vi "test_serialize_deserialize.vi"   [LabVIEW 2020, in "Optitrack.lvlib"]
doc: "Version 0.1"
uses:
  <vilib>/ADAS Record/CustomDataTypes/Optitrack/Optitrack.lvlib
  <vilib>/addons/_JKI Toolkits/Caraya/classes/Test/Test.lvclass
  <vilib>/addons/_JKI Toolkits/Caraya/classes/Assert/Assert.lvclass
  <vilib>/ADAS Record/CustomDataTypes/Optitrack/Process Data.ctl
  <vilib>/ADAS Record/CustomDataTypes/ADAS Generic/Serialize Data.vi
  <vilib>/ADAS Record/CustomDataTypes/ADAS Generic/NI_ADAS_Generic.lvlib
  <vilib>/ADAS Record/CustomDataTypes/ADAS Generic/Deserialize Data.vi
  Projects/NI AzDO/Mercedes-MPIC-201077/Record_MPIC3/mercedes-record-mpic3-201077/software-record-plugins/labview-2020/src/shared/TypeDef-Optitrack-RigidBody.ctl
  Projects/NI AzDO/Mercedes-MPIC-201077/Record_MPIC3/mercedes-record-mpic3-201077/software-record-plugins/labview-2020/src/shared/TypeDef-Optitrack-MarkerPoint.ctl
  Projects/NI AzDO/Mercedes-MPIC-201077/Record_MPIC3/mercedes-record-mpic3-201077/software-record-plugins/labview-2020/src/shared/TypeDef-Optitrack-MarkerSet.ctl
  Projects/NI AzDO/Mercedes-MPIC-201077/Record_MPIC3/mercedes-record-mpic3-201077/software-record-plugins/labview-2020/src/shared/TypeDef-Optitrack-LabeledMarker.ctl
  Projects/NI AzDO/Mercedes-MPIC-201077/Record_MPIC3/mercedes-record-mpic3-201077/software-record-plugins/labview-2020/src/shared/TypeDef-Optitrack-TrackedData.ctl
  Projects/NI AzDO/Mercedes-MPIC-201077/Record_MPIC3/mercedes-record-mpic3-201077/software-record-plugins/labview-2020/src/shared/TypeDef-Optitrack-FrameData.ctl
types:
  T1 = typedef "Optitrack.lvlib/Process Data.ctl" = cluster{"OptitrackFrame":T2}
  T2 = typedef "TypeDef-Optitrack-FrameData.ctl" = cluster{"# Labeled Markers":i32, "Frame":i32, "# Marker Sets":i32, "Relative Timestamp":dbl, "# Other Markers":i32, "# Rigid Bodies":i32, "# Skeletons":i32, "# Force Plates":i32, "# Devices":i32, "Timecode":u32, "Timecode Subframe":u32, "Mid Exposure Timestamp":u64, "Data Received Timestamp":u64, "Transmit Timestamp":u64, "Tracking Models Changed":bool, "Recording":bool, "Tracked Data":T3, "Statistics":cluster{"Dropped Frames":i32, "Frames Remaining":i32, "FPS":dbl}, "Frame Timestamp":timestamp}
  T3 = typedef "TypeDef-Optitrack-TrackedData.ctl" = cluster{"Labled Markers Data":T4[], "Marker Sets Data":T5[], "Rigid Bodies Data":T7[]}
  T4 = typedef "TypeDef-Optitrack-LabeledMarker.ctl" = cluster{"X":sgl, "Y":sgl, "Z":sgl, "Size":sgl, "Residual":sgl, "Parameters":i16, "ID":i32}
  T5 = typedef "TypeDef-Optitrack-MarkerSet.ctl" = cluster{"Marker Set Name":string, "Marker Points":T6[]}
  T6 = typedef "TypeDef-Optitrack-MarkerPoint.ctl" = cluster{"X":sgl, "Y":sgl, "Z":sgl}
  T7 = typedef "TypeDef-Optitrack-RigidBody.ctl" = cluster{"ID":i32, "Mean Error":sgl, "qw":sgl, "qx":sgl, "qy":sgl, "qz":sgl, "Tracked":bool, "x":sgl, "y":sgl, "z":sgl, "Rigid Body Name":string}
  T8 = typedef "NI_ADAS_Generic.lvlib/Process Data.ctl" = cluster{"Timestamp":timestamp, "Bus Channel":u16, "Byte Array":u8[]}
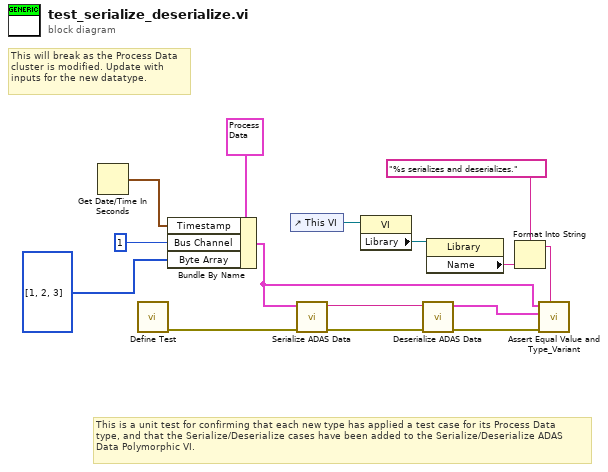
[diagram p0: block diagram]
diagram:
  # "This will break as the Process Data\ncluster is modified. Update with\ninputs for the new datatype."
  # "This is a unit test for confirming that each new type has applied a test case for its Process Data\ntype, and that the Serialize/Deserialize cases have been added to the Serialize/Deserialize ADAS\nData Polymorphic VI."
  n1 = Get Date/Time In Seconds() -> (seconds since 1Jan1904=w4:timestamp)
  n2 = call <vilib>:"Define Test.vi"() -> ("error out"=w10:errorcluster)  [unwired: 11 in]
  n3 = Bundle By Name(cluster=T1 {"OptitrackFrame"={"# Labeled Markers"=0, "Frame"=0, "# Marker Sets"=0, "Relative Timestamp"=0.0, "# Other Markers"=0, "# Rigid Bodies"=0, "# Skeletons"=0, "# Force Plates"=0, "# Devices"=0, "Timecode"=0, "Timecode Subframe"=0, "Mid Exposure Timestamp"=0, "Data Received Timestamp"=0, "Transmit Timestamp"=0, "Tracking Models Changed"=FALSE, "Recording"=FALSE, "Tracked Data"={"Labled Markers Data"=[], "Marker Sets Data"=[], "Rigid Bodies Data"=[]}, "Statistics"={"Dropped Frames"=0, "Frames Remaining"=0, "FPS"=0.0}, "Frame Timestamp"=timestamp(0 s since 1904-01-01)}} ("Process Data in"), "Timestamp"=w4, "Bus Channel"=u16 1, "Byte Array"=u8[] [1, 2, 3]) -> (w1:T1)
  n4 = control-ref of="This VI"() -> (w15:refnum<vi>)
  n5 = call-poly <vilib>:"Serialize ADAS Data.vi"("error in (no error)"=w10, "Process Data"=w1) -> ("error out"=w9:errorcluster, "Flat Data out"=w8:string)  [unwired: 8 in]
  n6 = property class="VI"(reference=w15) -> ("Library"=w14:refnum<vi>)  [unwired: 1 in, 2 out]
  n7 = call-poly <vilib>:"Deserialize ADAS Data.vi"("error in (no error)"=w9, "Flat Data in"=w8) -> ("error out"=w6:errorcluster, "Process Data out"=w7:T8)  [unwired: 8 in]
  n8 = property class="Library"(reference=w14) -> ("Name"=w12:string)  [unwired: 1 in, 2 out]
  n9 = Format Into String(format string="%s serializes and deserializes.", w12) -> (resulting string=w11:string)  [unwired: 2 in, 1 out]
  n10 = call <vilib>:"Assert Equal Value and Type_Variant.vi"("Label"=w11, "error in (no error)"=w6, "Y"=w7, "X"=w1) -> ()  [unwired: 7 in, 1 out]
